vi "Controller FOFB Configuration In to Out.vi"(11 "LNLS Control FOFB Configuration In":T3={"Status"=0, "Operation Mode"=enum."Manual Mode", "PID Horizontal Gain"=0.0, "PID Vertical Gain"=0.0, "PID Horizontal Integral Time"=0.0, "PID Vertical Integral Time"=0.0, "PID Horizontal Derivative Time"=0.0, "PID Vertical Derivative Time"=0.0, "Fast Command Enabled"=FALSE}) -> (3 "LNLS Control FOFB Configuration Out":T1)   [LabVIEW 2011, in "Controller VIs.lvlib"]
uses:
  Controller VIs.lvlib
  Types Definitions/Type Control FOFB Configuration In.ctl
  Types Definitions/Type Operation Mode State.ctl
  Types Definitions/Type Control FOFB Configuration Out.ctl
  Type Definitions.lvlib
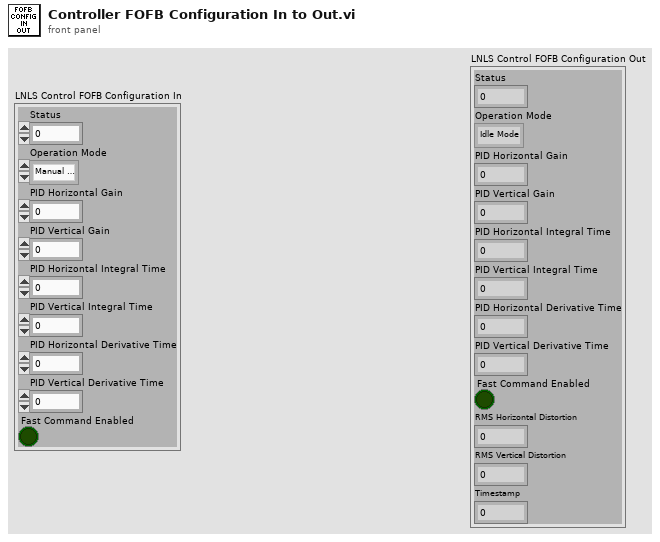
[diagram p1: front panel]
types:
  T1 = typedef "Type Definitions.lvlib/Type Control FOFB Configuration Out.ctl" = cluster{"Status":u16, "Operation Mode":T2, "PID Horizontal Gain":sgl, "PID Vertical Gain":sgl, "PID Horizontal Integral Time":sgl, "PID Vertical Integral Time":sgl, "PID Horizontal Derivative Time":sgl, "PID Vertical Derivative Time":sgl, "Fast Command Enabled":bool, "RMS Horizontal Distortion":dbl, "RMS Vertical Distortion":dbl, "Timestamp":dbl}
  T2 = typedef "Type Definitions.lvlib/Type Operation Mode State.ctl" = enum8{"Idle Mode", "Manual Mode", "FOFB Mode", "RMM Mode"}
  T3 = typedef "Type Definitions.lvlib/Type Control FOFB Configuration In.ctl" = cluster{"Status":u16, "Operation Mode":T2, "PID Horizontal Gain":sgl, "PID Vertical Gain":sgl, "PID Horizontal Integral Time":sgl, "PID Vertical Integral Time":sgl, "PID Horizontal Derivative Time":sgl, "PID Vertical Derivative Time":sgl, "Fast Command Enabled":bool}
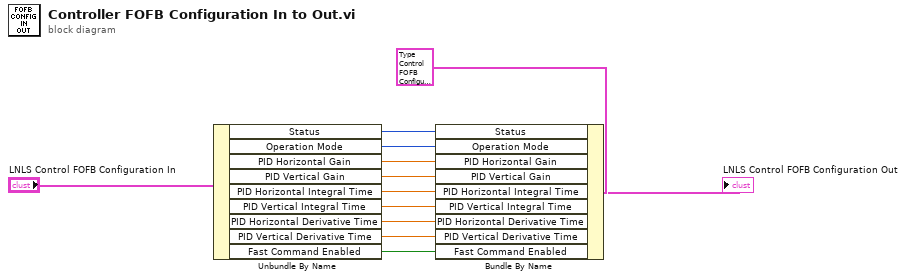
[diagram p0: block diagram]
diagram:
  n1 = Unbundle By Name("LNLS Control FOFB Configuration In") -> ("Status"=w12:u16, "Operation Mode"=w11:T2, "PID Horizontal Gain"=w10:sgl, "PID Vertical Gain"=w9:sgl, "PID Horizontal Integral Time"=w8:sgl, "PID Vertical Integral Time"=w7:sgl, "PID Horizontal Derivative Time"=w6:sgl, "PID Vertical Derivative Time"=w5:sgl, "Fast Command Enabled"=w1:bool)
  n2 = Bundle By Name(cluster=T1 {"Status"=0, "Operation Mode"=enum."FOFB Mode", "PID Horizontal Gain"=0.0, "PID Vertical Gain"=0.0, "PID Horizontal Integral Time"=0.0, "PID Vertical Integral Time"=0.0, "PID Horizontal Derivative Time"=0.0, "PID Vertical Derivative Time"=0.0, "Fast Command Enabled"=FALSE, "RMS Horizontal Distortion"=0.0, "RMS Vertical Distortion"=0.0, "Timestamp"=0.0} ("LNLS Control FOFB Configuration Out"), "Status"=w12, "Operation Mode"=w11, "PID Horizontal Gain"=w10, "PID Vertical Gain"=w9, "PID Horizontal Integral Time"=w8, "PID Vertical Integral Time"=w7, "PID Horizontal Derivative Time"=w6, "PID Vertical Derivative Time"=w5, "Fast Command Enabled"=w1) -> (→"LNLS Control FOFB Configuration Out":T1)
